vi "generatore_rettangolare_-1_1.vi"(0 "f0 (frequenza base) [Hz]":dbl min=0.0, 1 "Ap (ampiezza di picco)":dbl min=0.0, 2 "Tc (periodo di campionamento) [s]":dbl min=0.0, 3 "Ta (tempo di analisi) [s]":dbl min=0.0, 4 "Duty Cycle (onda rettangolare)":dbl min=0.0 max=1.0, 5 "Phi (fase iniziale) [rad]":dbl, 8 "DC Offset":dbl) -> (7 "Waveform Graph":waveform(dbl)(graph))   [LabVIEW 2009]
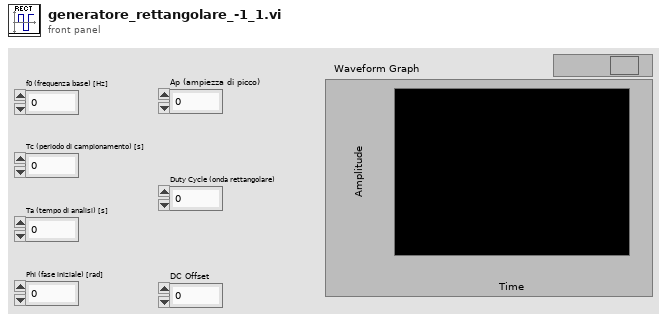
[diagram p1: front panel]
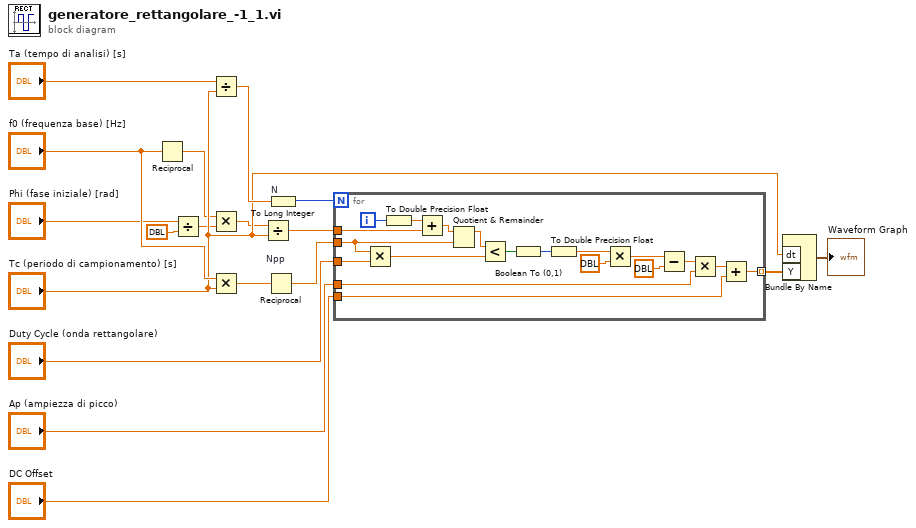
[diagram p0: block diagram]
diagram:
  n1 = Reciprocal(x="f0 (frequenza base) [Hz]") -> (1/x=w5:dbl)
  n2 = Divide(x="Phi (fase iniziale) [rad]", y=dbl ?) -> (x/y=w6:dbl)
  n3 = Divide(x="Ta (tempo di analisi) [s]", y="Tc (periodo di campionamento) [s]") -> (x/y=w11:dbl)
  n4 = Multiply(x=w5, y=w6) -> (x*y=w4:dbl)
  n5 = Multiply(x="f0 (frequenza base) [Hz]", y="Tc (periodo di campionamento) [s]") -> (x*y=w17:dbl)
  n6 = Divide(x=w4, y="Tc (periodo di campionamento) [s]") -> (x/y=w2:dbl)
  n7 = Reciprocal "Npp"(x=w17) -> (1/x=w18:dbl)
  n8 = To Long Integer "N"(number=w11) -> (32bit integer=w12:i32)
  n9 = for {
    N: w12 -> [_]
    tunnel: "DC Offset" -> [w37]
    tunnel: "Ap (ampiezza di picco)" -> [w20]
    tunnel: "Duty Cycle (onda rettangolare)" -> [w35]
    tunnel: [w36] -> w9 mode=indexing
    tunnel: w18 -> [w34]
    tunnel: w2 -> [w24]
    i -> [w33]
    n10 = Multiply(x=w34, y=w35) -> (x*y=w29:dbl)
    n11 = To Double Precision Float(number=w33) -> (double precision float=w32:dbl)
    n12 = Add(x=w32, y=w24) -> (x+y=w31:dbl)
    n13 = Quotient & Remainder(x=w31, y=w34) -> (x-y*floor(x/y)=w30:dbl)  [unwired: 1 out]
    n14 = Less?(x=w30, y=w29) -> (x < y?=w28:bool)
    n15 = Boolean To (0,1)(Boolean=w28) -> (0, 1=w27:i16)
    n16 = To Double Precision Float(number=w27) -> (double precision float=w26:dbl)
    n17 = Multiply(x=w26, y=dbl ?) -> (x*y=w25:dbl)
    n18 = Subtract(x=w25, y=dbl ?) -> (x-y=w21:dbl)
    n19 = Multiply(x=w21, y=w20) -> (x*y=w19:dbl)
    n20 = Add(x=w19, y=w37) -> (x+y=w36:dbl)
  }
  n21 = Bundle By Name("dt"="Tc (periodo di campionamento) [s]", "Y"=w9) -> (→"Waveform Graph":waveform(dbl))  [unwired: 1 in]
